vi "Bind Terminal Visibility.vi"(5 "Datum Type (Boolean)":variant, 6 "Inverse Binding Logic?":bool, 7 "Initial Visible State (T)":bool=TRUE, 8 "error in (no error)":errorcluster, 9 "Datum Name (\"\"=Use Control Label)":string, 10 "Ctl Refnum":refnum<vi>, 11 "IViewable in":refnum<class "IViewable.lvclass">) -> (0 "error out":errorcluster, 3 "IViewable out":refnum<class "IViewable.lvclass">)   [LabVIEW 2020, in "IViewable.lvlib" / "IViewable.lvclass"]
doc: "Bind the visible state of a control terminal (control or indicator) to a published Boolean or Numeric datum. Specify the logical relationship between datum vale and terminal visibility by wiring the optional input terminals.\n\nDefault for Boolean:\nPublished TRUE = Visible\nPublished FALSE = Hidden\n\nDefault for Numeric:\nPublised value greater than 0 = Visible\nPublished value NOT greater than 0 = Hidden"
uses:
  IViewable.lvclass
  IViewable.lvclass/IViewable.ctl
  mva-core/Source/IMediator/SubscriptionRequest/SubscriptionRequest.lvclass
  mva-core/Source/IObserver/IObserver Messages/Subscribe Msg/Subscribe Msg.lvclass
  <vilib>/ActorFramework/Actor/Actor.lvclass
  mva-core/Source/IMediator/ISubscriptionPolicy/ISubscriptionPolicy.lvclass
  <vilib>/Utility/Data Type/NI_Data Type.lvlib
  composed-transport/Source/Concrete/TerminalVisibilityBinding/TerminalVisibilityBinding.lvclass
  mva-core/Source/SubscriptionPolicy/BasicSubscription/BasicSubscription.lvclass
  C:/Program Files/National Instruments/LabVIEW 2020/vi.lib/ActorFramework/Actor/Actor.lvclass
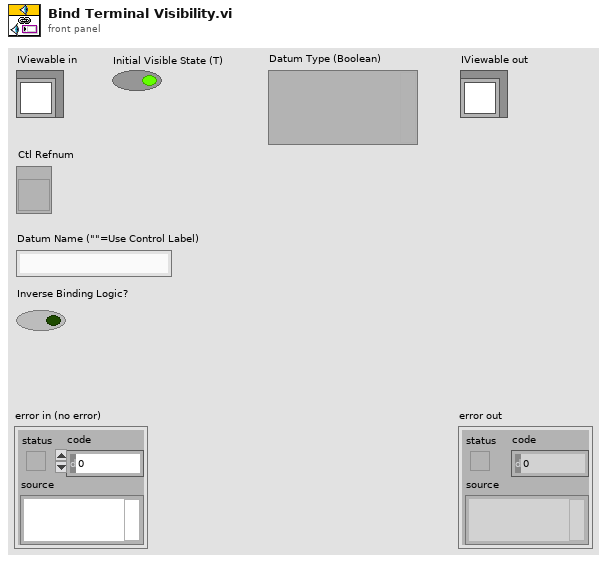
[diagram p1: front panel]
types:
  T1 = typedef "NI_Data Type.lvlib/Data Type.ctl" = enum8{"Invalid Type", "Void", "I8", "I16", "I32", "I64", "U8", "U16", "U32", "U64", "Single Float", "Double Float", "Extended Float", "Single Complex", "Double Complex", "Extended Complex", "Enum U8", "Enum U16", "Enum U32", "Enum U64", "Single Float With Unit", "Double Float With Unit", "Extended Float With Unit", "Single Complex with Unit", "Double Complex with Unit", "Extended Complex with Unit", "Boolean", "String", "Path", "Picture", "Tag", "Array", "Cluster", "Variant", "LV Variant", "Waveform", "Timestamp", "Digital Waveform", "Digital Data", "ExpressData", "Refnum", "External Data", "VI", "Poly VI", "LabVIEW Class Instance", "Fixed Point", "Set Collection", "Map Collection"}
  T2 = typedef "IMediator.lvlib/ISubscriptionPolicy.lvclass/ISubscriptionPolicy Reference.ctl" = refnum<data-value>
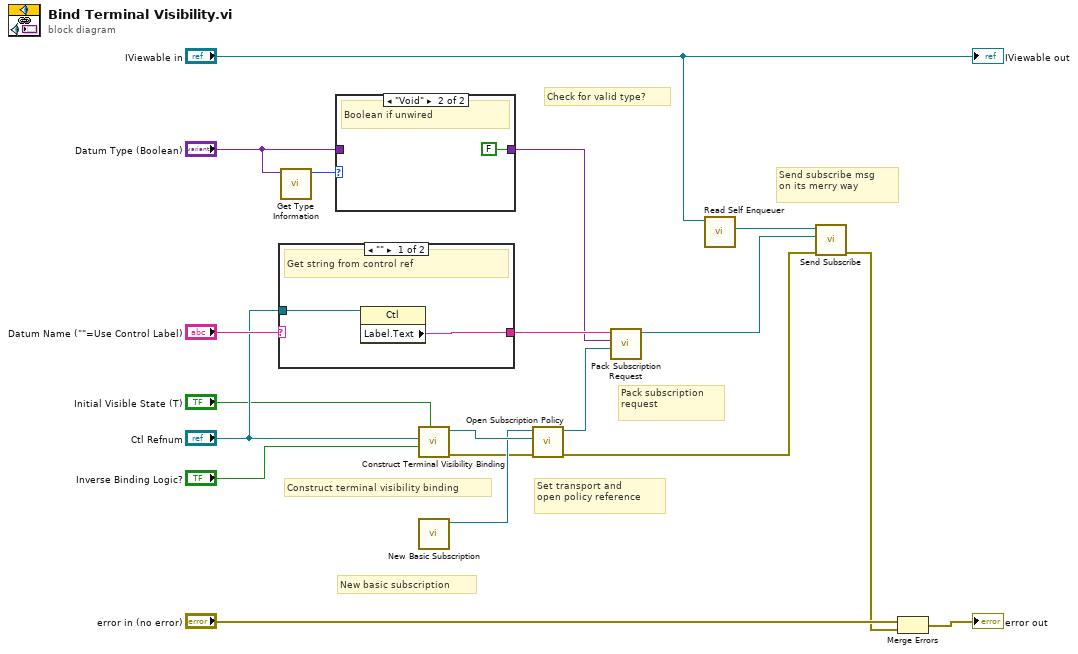
[diagram p0: block diagram]
diagram:
  # "Check for valid type?"
  # "New basic subscription"
  # "Set transport and\nopen policy reference"
  # "Send subscribe msg\non its merry way"
  # "Pack subscription\nrequest"
  # "Construct terminal visibility binding"
  n1 = case shown="\"\"" "Datum Name (\"\"=Use Control Label)" {
    selector: "Datum Name (\"\"=Use Control Label)" -> [_ w22]
    tunnel: [w20 w22] -> w12
    tunnel: "Ctl Refnum" -> [w21 _]
    frame "" {
      # "Get string from control ref"
      n2 = property class="Ctl"(reference=w21) -> ("Label.Text"=w20:string)  [unwired: 1 in, 2 out]
    }
    frame Default {
      # "Use string wired to input terminal"
    }
  }
  n3 = call <vilib>:"Get Type Information.vi"("variant"="Datum Type (Boolean)") -> ("type"=w8:T1)  [unwired: 6 in, 4 out]
  n4 = case shown="\"Void\"" w8 {
    tunnel: [w23 FALSE] -> w6
    tunnel: "Datum Type (Boolean)" -> [w23 _]
    frame Default {
      # "Only Boolean and Numeric\nproduce valid subscription"
      # "Use wired type"
    }
    frame "Void" {
      # "Boolean if unwired"
    }
  }
  n5 = call "Construct Terminal Visibility Binding.vi"("Initial Visible State (T)"="Initial Visible State (T)", "Inverse Visible Logic? (F)"="Inverse Binding Logic?", "Ctl Refnum"="Ctl Refnum") -> ("error out"=w4:errorcluster, "TerminalVisibilityBinding"=w10:refnum<class "TerminalVisibilityBinding.lvclass">)  [unwired: 7 in]
  n6 = call "New Basic Subscription.vi"() -> ("BasicSubscription Out"=w9:refnum<class "BasicSubscription.lvclass">)  [unwired: 11 in]
  n7 = call "Open Subscription Policy.vi"("error in (no error)"=w4, "Transport"=w10, "SubscriptionPolicy"=w9) -> ("error out"=w1:errorcluster, "Subscription Policy"=w2:T2)  [unwired: 7 in]
  n8 = call "Pack Subscription Request.vi"("Subscription Policy"=w2, "Type"=w6, "Datum Name"=w12) -> ("SubscriptionRequest"=w16:refnum<class "SubscriptionRequest.lvclass">)  [unwired: 7 in, 1 out]
  n9 = call <vilib>:"Read Self Enqueuer.vi"("Actor"="IViewable in") -> ("Self Enqueuer"=w17:refnum<class "Message Enqueuer.lvclass">)  [unwired: 10 in]
  n10 = call "Send Subscribe.vi"("error in (no error)"=w1, "SubscriptionRequest"=w16, "Message Enqueuer"=w17) -> ("error out"=w14:errorcluster)  [unwired: 7 in, 1 out]
  n11 = Merge Errors("error in (no error)", w14) -> (→"error out":errorcluster)
  "IViewable out" <- "IViewable in"
